vi "image recorder main panel.vi"() -> ()   [LabVIEW 2013]
uses:
  <vilib>/Utility/error.llb/DialogType.ctl
  Image-Stack-Compressor/StackWriterWrapper/LV code/StackWriterWrapper.lvlib
  <vilib>/ptbypt/NI_PtbyPt.lvlib
panel:
  out "frame add time":u32
  out "last loop time":u32
  in  "left of screen":string="air inlet"
  in  "bottom of screen":string="CS"
  in  "top of screen":string="back of box (y = 0)"
  in  "central region (frac)":dbl caption="central region for placement\nsize (fraction of full screen)"
  out "loop time":u32
  in  "max Background Compression Threads":i32=4
  in  "maxBytesToWrite":u64=1950000000 format="%.2p"
  in  "limit file size?":bool
  out "notes last updated":timestamp format="%<%I:%M %p\n%d/%m/%y>T"
  in  "notes":string
  out "avg frame rate (fps)":dbl
  out "total loop\nwith delay":u32
  out "delay time":dbl
  in  "auto-set":bool
  out "numToWrite":i32(slide) scale=0.0..10.0
  out "numToCompress":i32(slide)=1 scale=0.0..10.0
  out "loop too fast":bool
  in  "min loop time (ms)":u32
  out "timing report":string="-\n  name: adding frame to stack\n  ncalls: 72\n  totaltime: 0.298202\n  maxtime: 0.00436328\n  mintime: 0.00225001\n  avg time: 0.00414169\n  numblowntics: 0\n-\n  name: cloning image\n  ncalls: 72\n  totaltime: 0.24642\n  maxtime: 0.00378184\n  mintime: 0.0017782\n  avg time: 0.0034225\n  numblowntics: 0\n-\n  name: compressing a frame\n  ncalls: 72\n  totaltime: 1.94123\n  maxtime: 0.0403699\n  mintime: 0.0239481\n  avg time: 0.0269615\n  numblowntics: 0\n-\n  name: creating save description\n  ncalls: 1\n  totaltime: 6.19014e-005\n  maxtime: 6.19014e-005\n  mintime: 6.19014e-005\n  avg time: 6.19014e-005\n  numblowntics: 0\n-\n  name: deleting written stack from memory\n  ncalls: 1\n  totaltime: 0.00222322\n  maxtime: 0.00222322\n  mintime: 0.00222322\n  avg time: 0.00222322\n  numblowntics: 0\n-\n  name: writing a stack to disk\n  ncalls: 1\n  totaltime: 0.0259505\n  maxtime: 0.0259505\n  mintime: 0.0259505\n  avg time: 0.0259505\n  numblowntics: 0\ncxcore: 1.0.0, cv: 1.0.0\n\n"
  out "stack destination":string="C:\\data\\test\\t10\\n#n#n#n\\CS(CS)\\2011\\09\\14\\1334\\CS@CS@t10@n#n#n#n@30.mmf"
  out "stackwriter pointer":u32=314603384
  out "loop iteration":i32=23494
  out "error out":errorcluster
  out "maximum loop time":u32
  out "average loop time":dbl format="%.2p"
  in  "max stack size":dbl=1.99
  out "GB written":dbl format="%.2f"
  out "max file size in GB":u64=8589934591
  out "MB written":i32
  out "average time to compress a frame":dbl format="%#_3p"
  out "average time to add a frame to stack":dbl format="%#_3p"
  out "average time to write a stack":dbl format="%#_3p"
  out "elapsed time(s)":dbl
  in  "anticipated frame rate":dbl=30.0
  in  "lgDimMinSize":i32=5
  in  "keyFrameInterval":i32=90
  in  "smallDimMinSize":i32=3
  in  "thresholdAboveBackground":i32=7
  out "buffer number":u32
  in  "base directory":path=path "C:/data/test"
  out "filename":string="CS@CS@t10@n#n#n#n@30"
  out "data directory":path=path "C:/data/test/t10/n#n#n#n/CS(CS)/2011/09/14/1334"
  in  "setup camera?":bool
  in  "STOP PROGRAM":bool
  in  "STOP ACQUISITION":bool
  in  "MAKE DIRECTORIES":bool
  in  "START ACQUISITION":bool
  in  "use ROI":bool
  in  "region of interest":cluster{"x0":u32, "y0":u32, "w":u32, "h":u32}={"x0"=0, "y0"=0, "w"=5000, "h"=5000}
  in  "Acquisiton Time (s)":dbl=660.0
  in  "update image every __ ms":u16=500
  out "Camera Image":T1(plugin-control)
  in  "set all control values as default":bool
  out "GAL4 Line":string="CS"
  in  "Experiment Description":T2={"GAL4 Line / Line A / Genotype"="CS", "UAS-Effector Line / Line B"="", "Experiment Type"=enum."olfaction", "Stimulus Descriptions"=[{"Stimulus Modulation"=enum."Spatial", "stimulant"="co2", "hi"=5, "lo"=0, "period"=20, "Modulation Detail"=enum."LinearX", "unit"="pct", "period_unit"="cm", "additional description"=enum."none", "description"=""}], "other name"="", "Training/Habituation Pre Exposure"={"CS"="", "UCS"="", "Training Protocol"="", "Training ID Code"="", "Training Type"=enum."none (no directory)"}}
  # "MMF compression settings"
  # "to reset to actual defaults, delete file\nimage recorder main panel ctl values.dflt"
  # "debugging stuff"
  # "X"
  # "lady gaga convention: when gradient is forward odor 1 \nhas minimum in lo field and maximum in hi field"
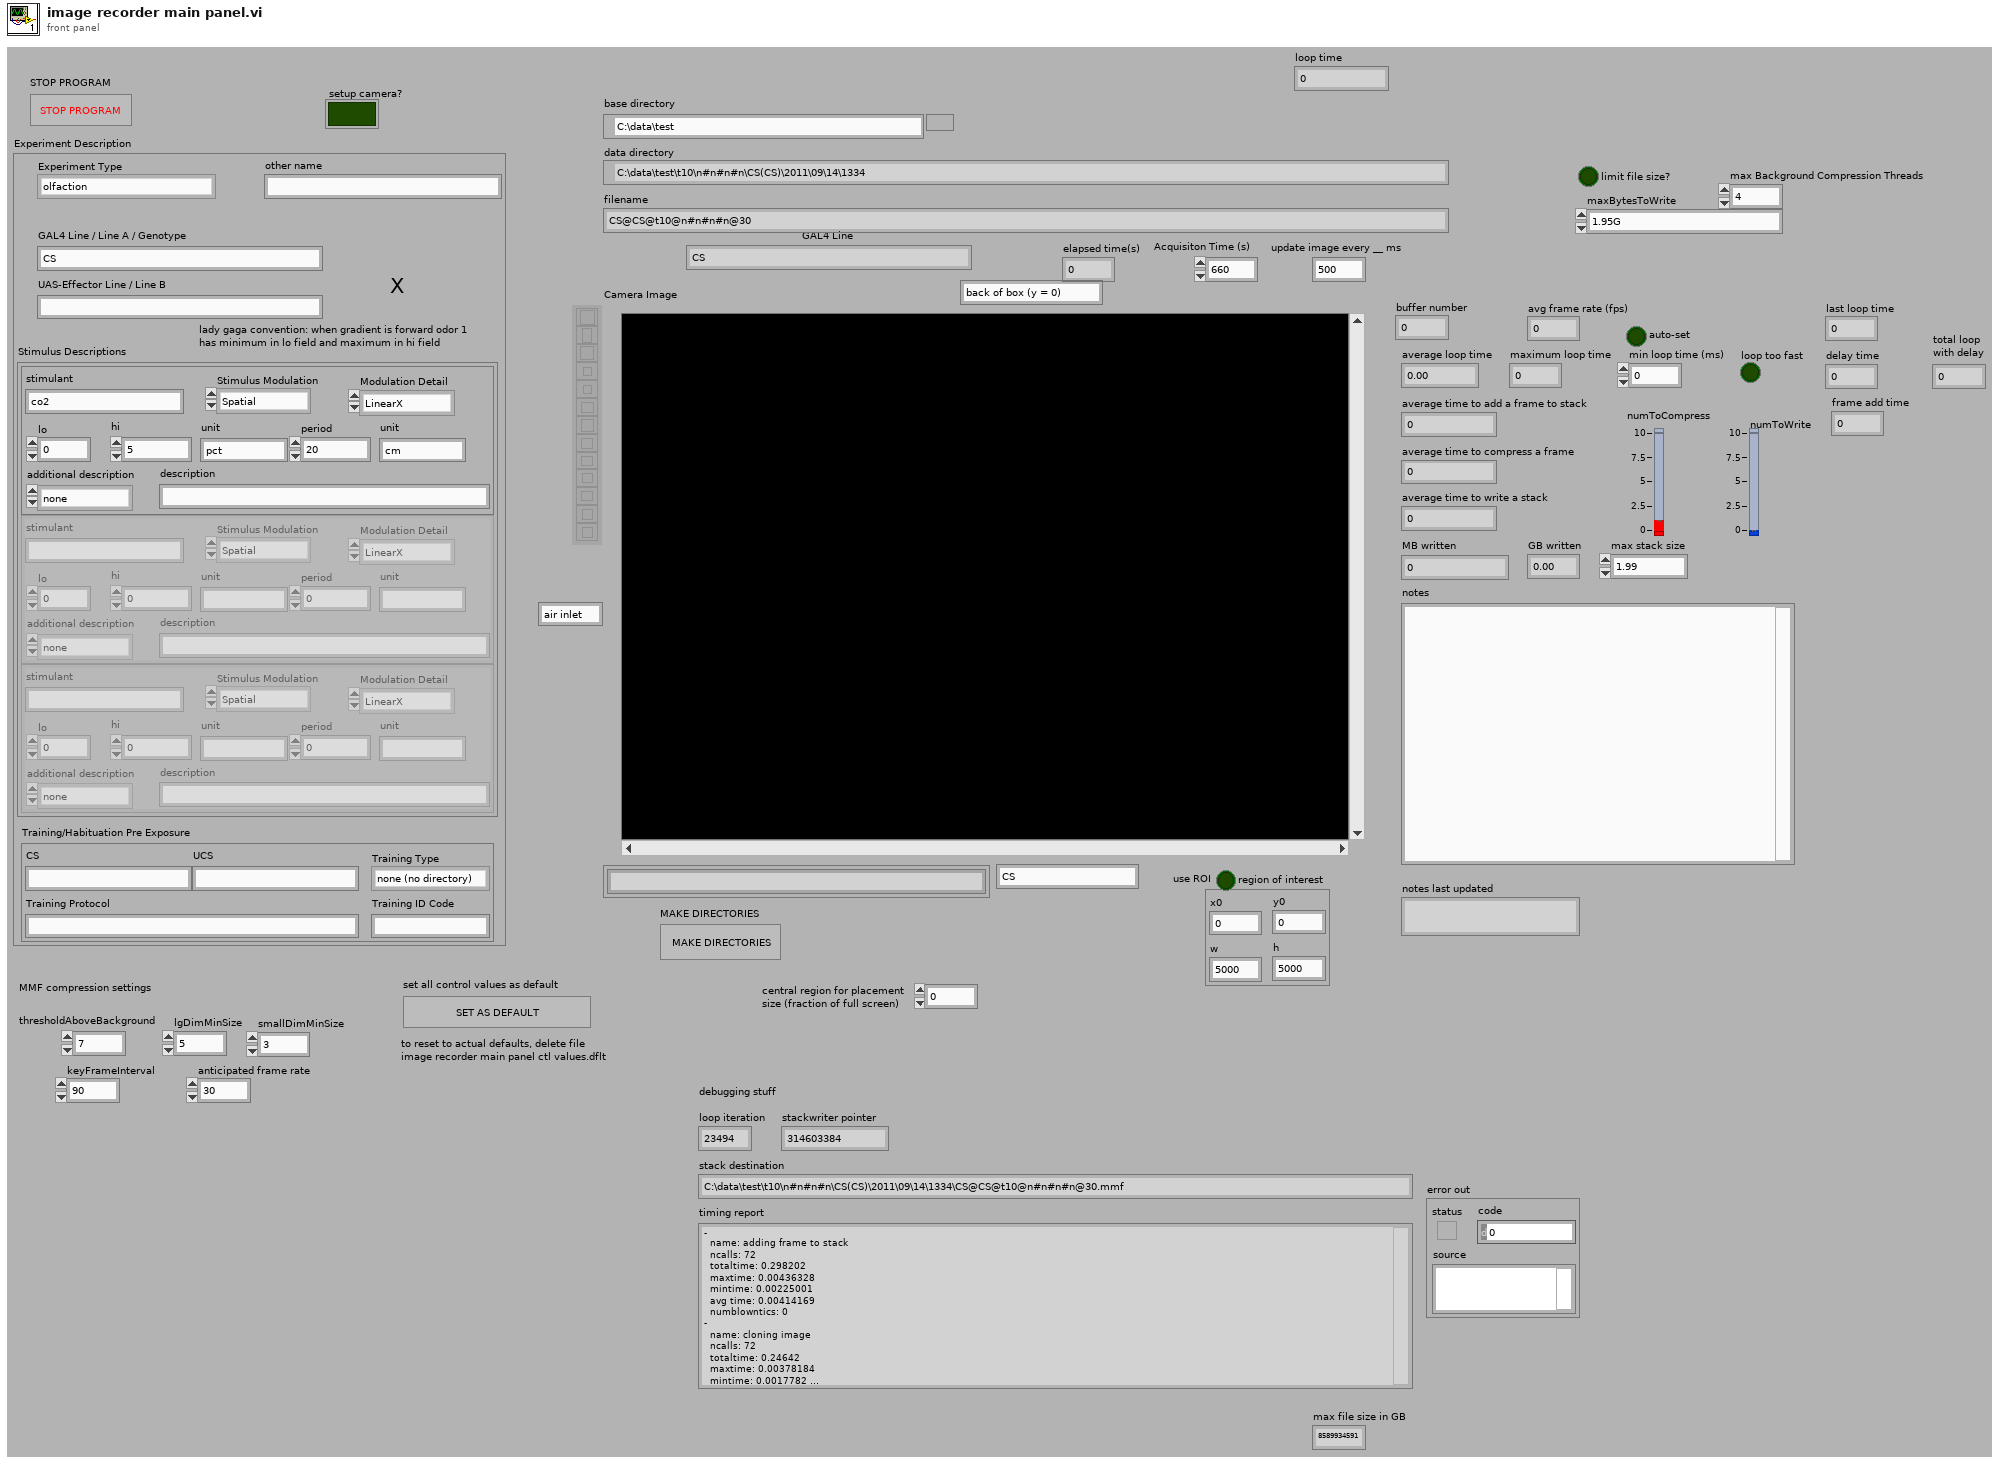
[diagram p1: front panel]
types:
  T1 = typedef "IMAQ Image.ctl" = refnum<image>
  T2 = cluster{"GAL4 Line / Line A / Genotype":string, "UAS-Effector Line / Line B":string, "Experiment Type":enum16{"other", "olfaction", "phototaxis", "chemotaxis", "thermotaxis", "multi sensory"}, "Stimulus Descriptions":cluster{"Stimulus Modulation":enum16{"Spatial", "Temporal", "Constant", "Other"}, "stimulant":string, "hi":u16, "lo":u16, "period":u16, "Modulation Detail":enum16{"LinearX", "LinearY", "Triangle", "Sine", "Square", "AngledX", "AngledY"}, "unit":string, "period_unit":string, "additional description":enum16{"none", "append", "replace"}, "description":string}[], "other name":string, "Training/Habituation Pre Exposure":cluster{"CS":string, "UCS":string, "Training Protocol":string, "Training ID Code":string, "Training Type":enum16{"none (no directory)", "untrained", "trained"}}}
  T3 = typedef "DialogType.ctl" = u16
  T4 = typedef "IMAQdx.ctl" = refnum<k21>
  T5 = cluster{"Aquisition Type":enum16{"IMAQ", "IMAQdx", "AVI", "MMF", "STACK"}, "Interface Name":string, "use roi":bool, "ROI":cluster{"left":u16, "top":u16, "width":u16, "height":u16}, "camera name":T4, "AVI Path":path, "mmf path":path, "stub":string, "Field Width (0 disables 0 padding)":u8, "extension":string, "inter-frame interval (ms)":dbl}
  T6 = typedef "AviRefnum.ctl" = refnum<k1>
  T7 = cluster{"Aquisition Type":enum16{"IMAQ", "IMAQdx", "AVI", "MMF", "STACK"}, "IMAQ Session Out":refnum<k11>, "imaqdx session":T4, "AVI parameters":cluster{"Avi Refnum ":T6, "inter-frame interval (ms)":dbl}, "mmf parameters":cluster{"mmf pointer":u32, "inter-frame interval (ms)":dbl}, "stack read info":cluster{"file stub":string, "format string":string, "extension":string, "inter-frame interval (ms)":dbl}, "camera image":T1, "camera image is 8 bit":bool, "8 bit camera image":T1}
  T8 = enum16{"Reset Table", "Get Values", "Add Value", "Get Table", "Get Spreadsheet", "set stack writer"}
  T9 = enum16{"open", "replace", "create", "open or create", "replace or create", "replace or create with confirmation"}
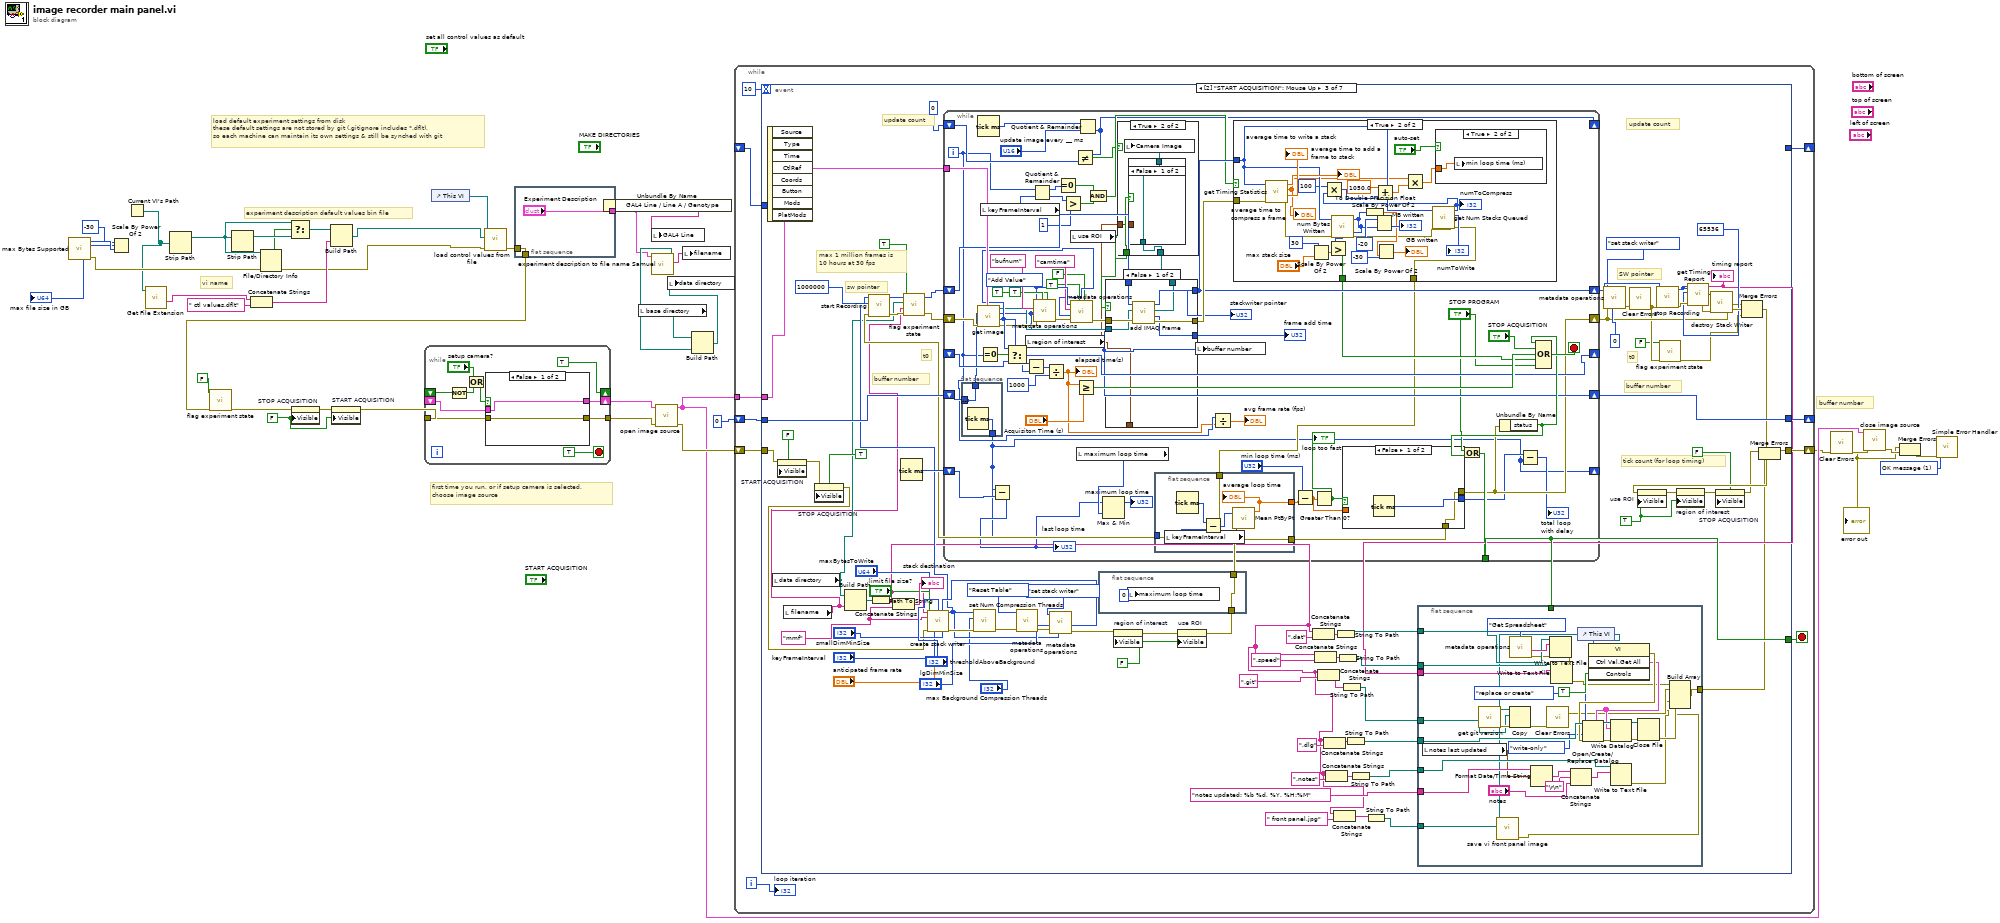
[diagram p0: block diagram]
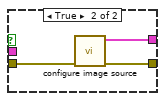
[diagram p2: hidden frame]
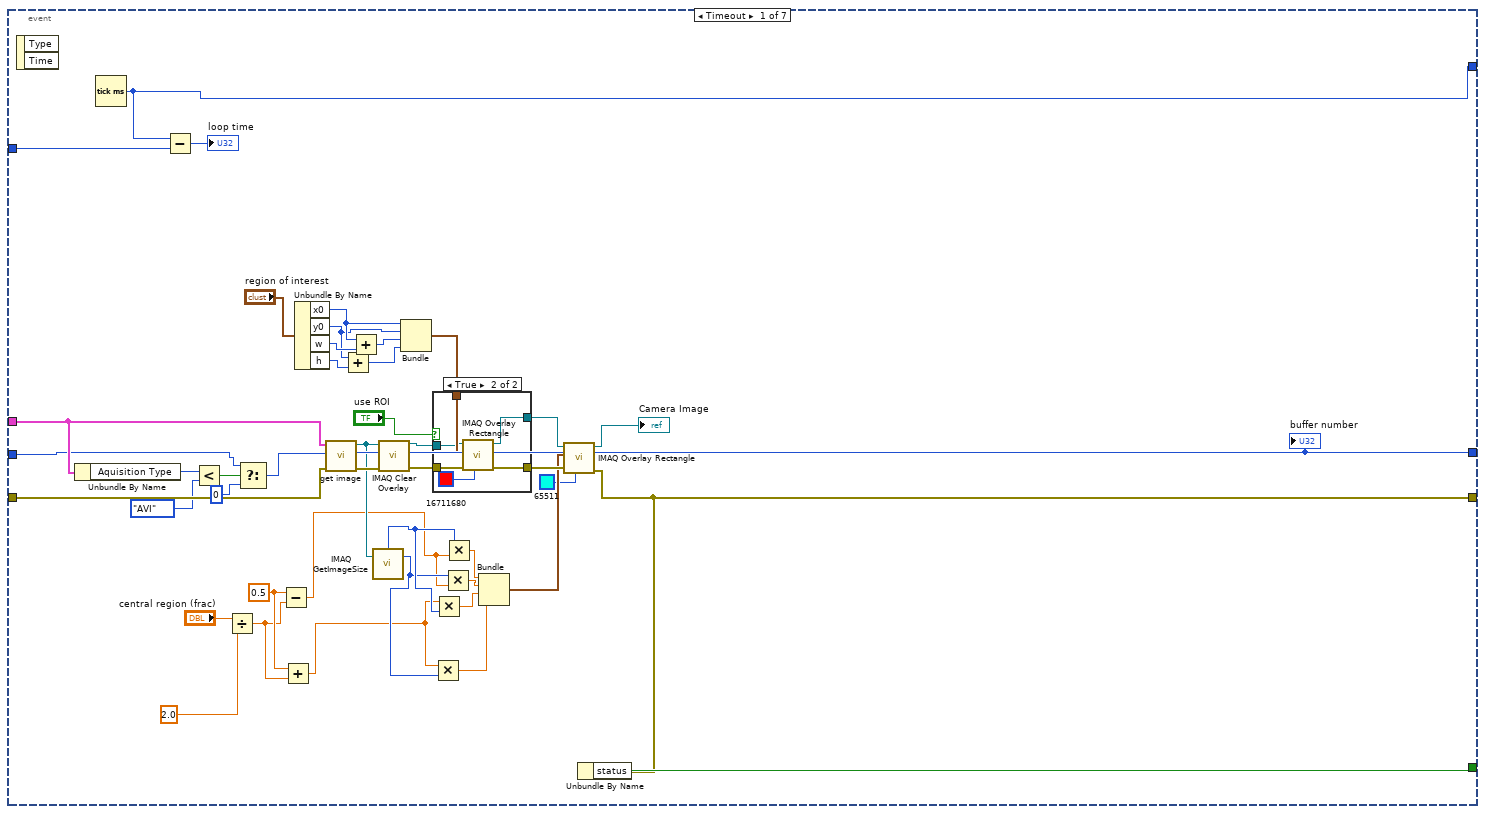
[diagram p3: hidden frame]
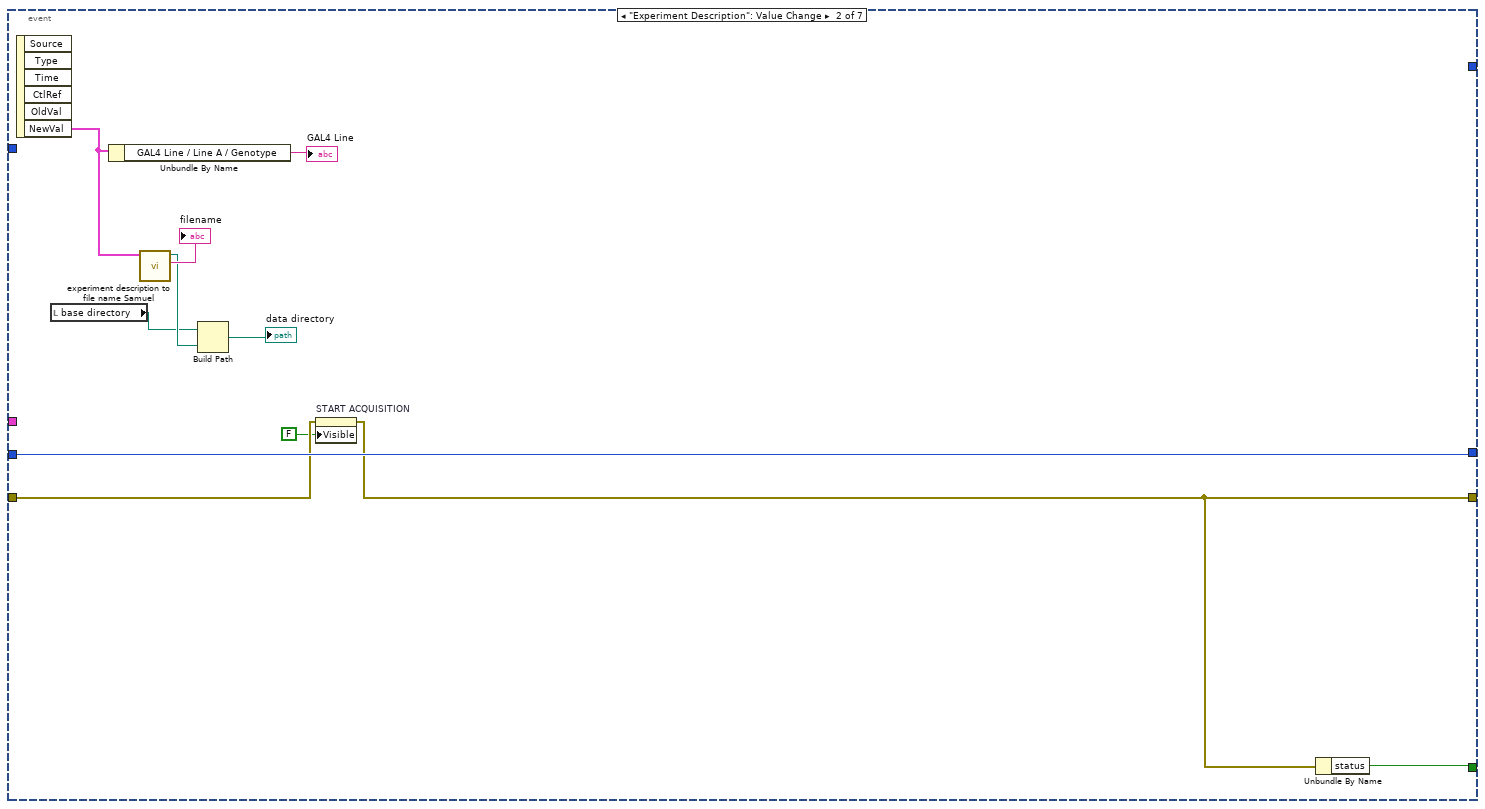
[diagram p5: hidden frame]
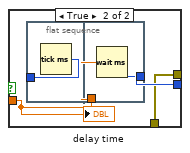
[diagram p6: hidden frame]
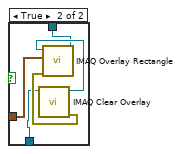
[diagram p8: hidden frame]
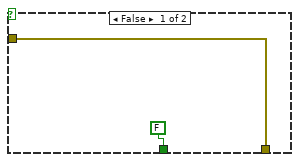
[diagram p9: hidden frame]
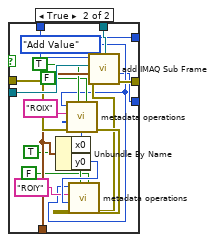
[diagram p11: hidden frame]
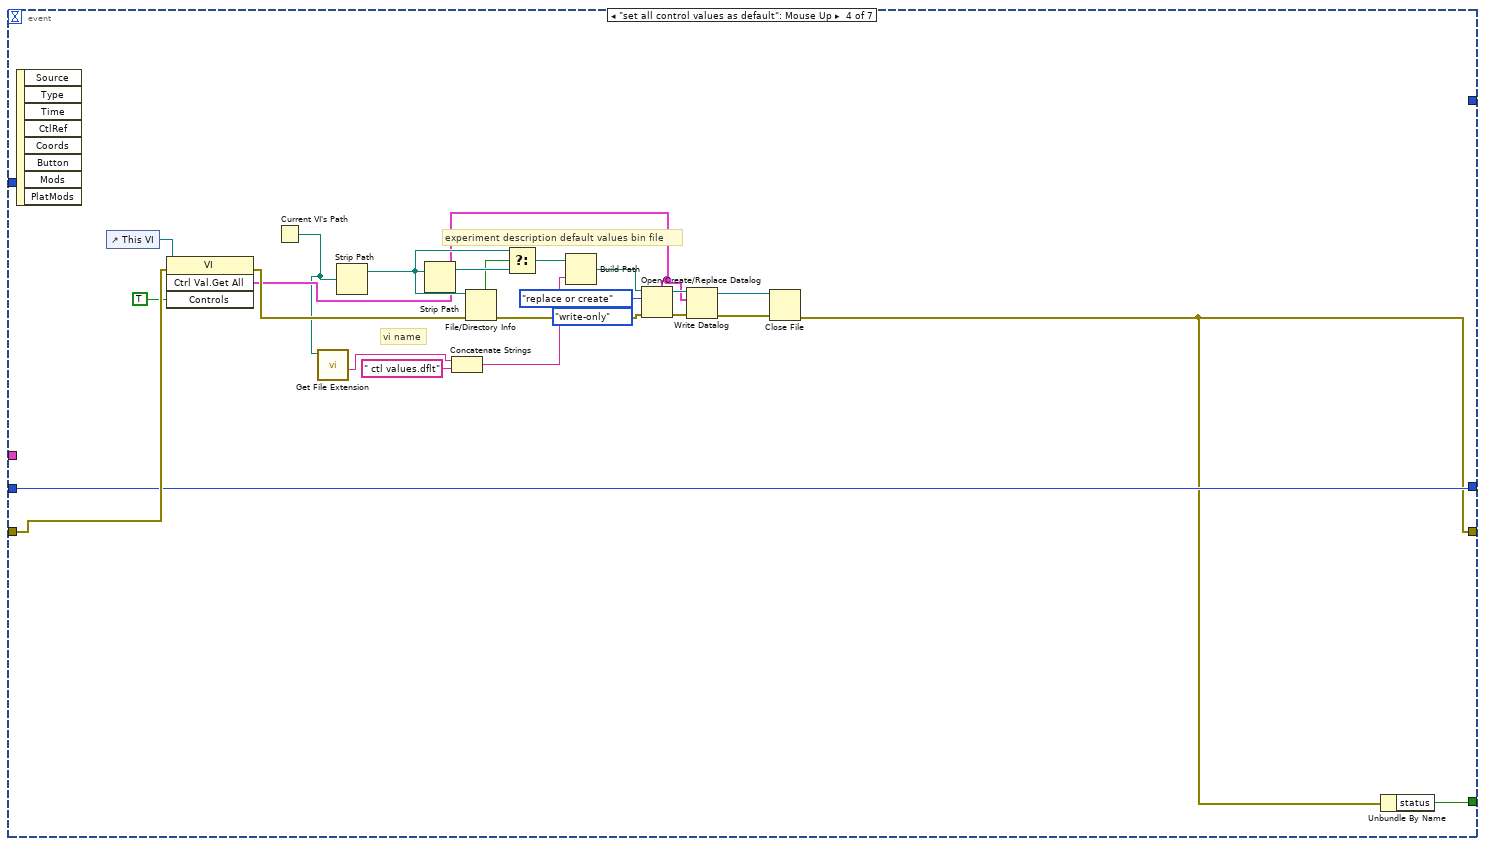
[diagram p12: hidden frame]
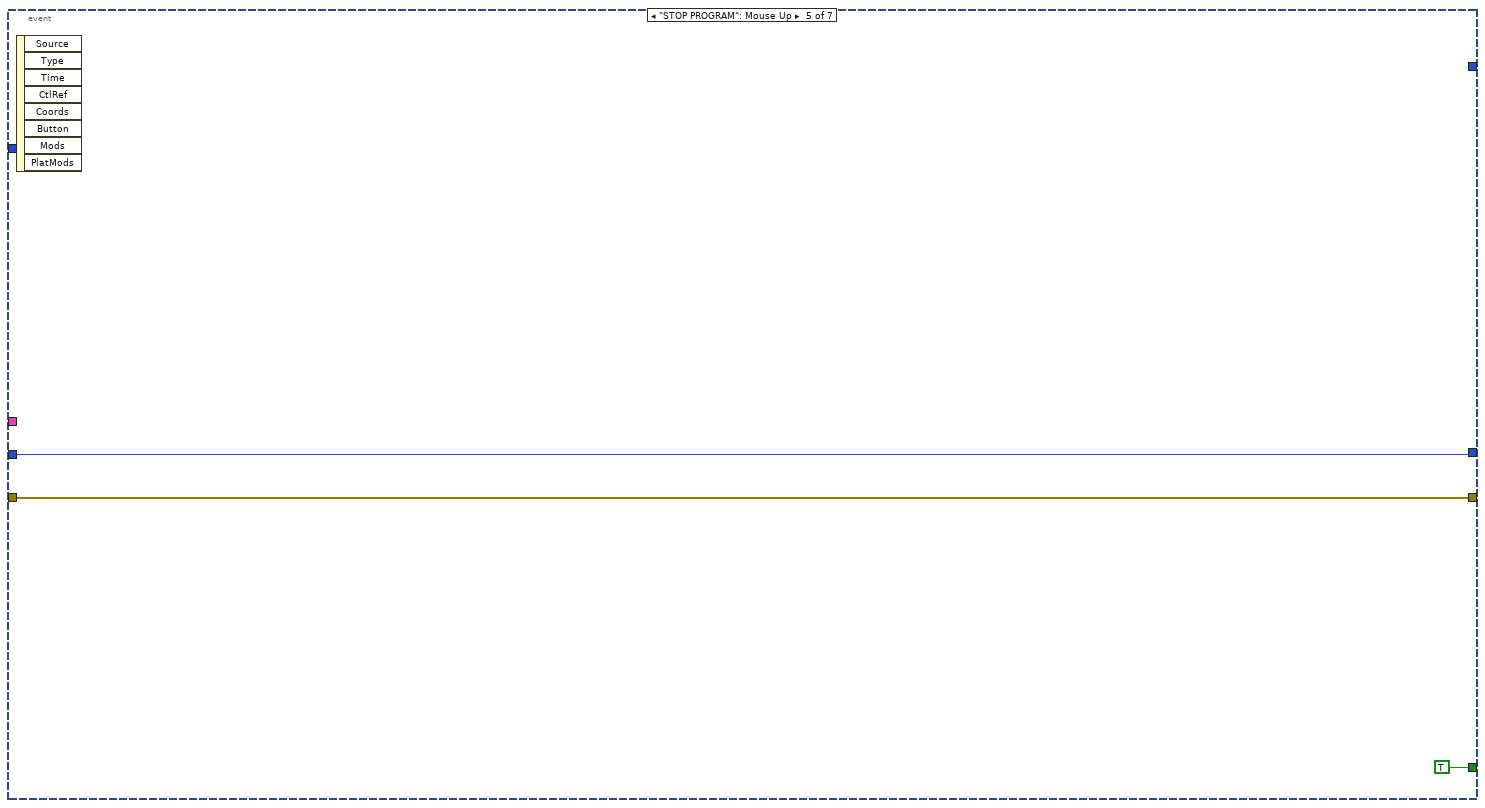
[diagram p13: hidden frame]
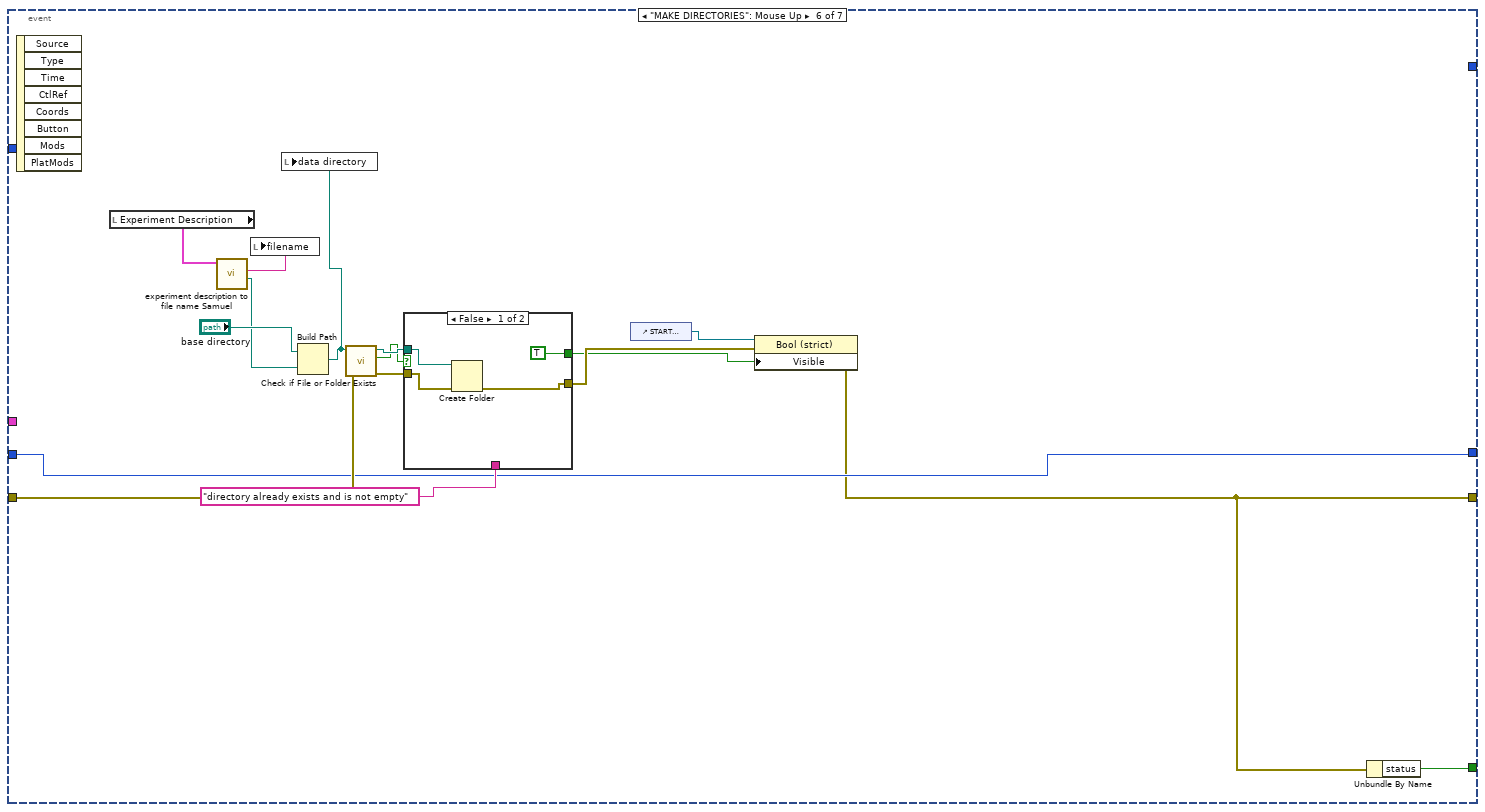
[diagram p14: hidden frame]
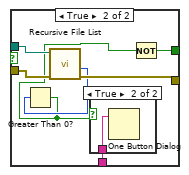
[diagram p15: hidden frame]
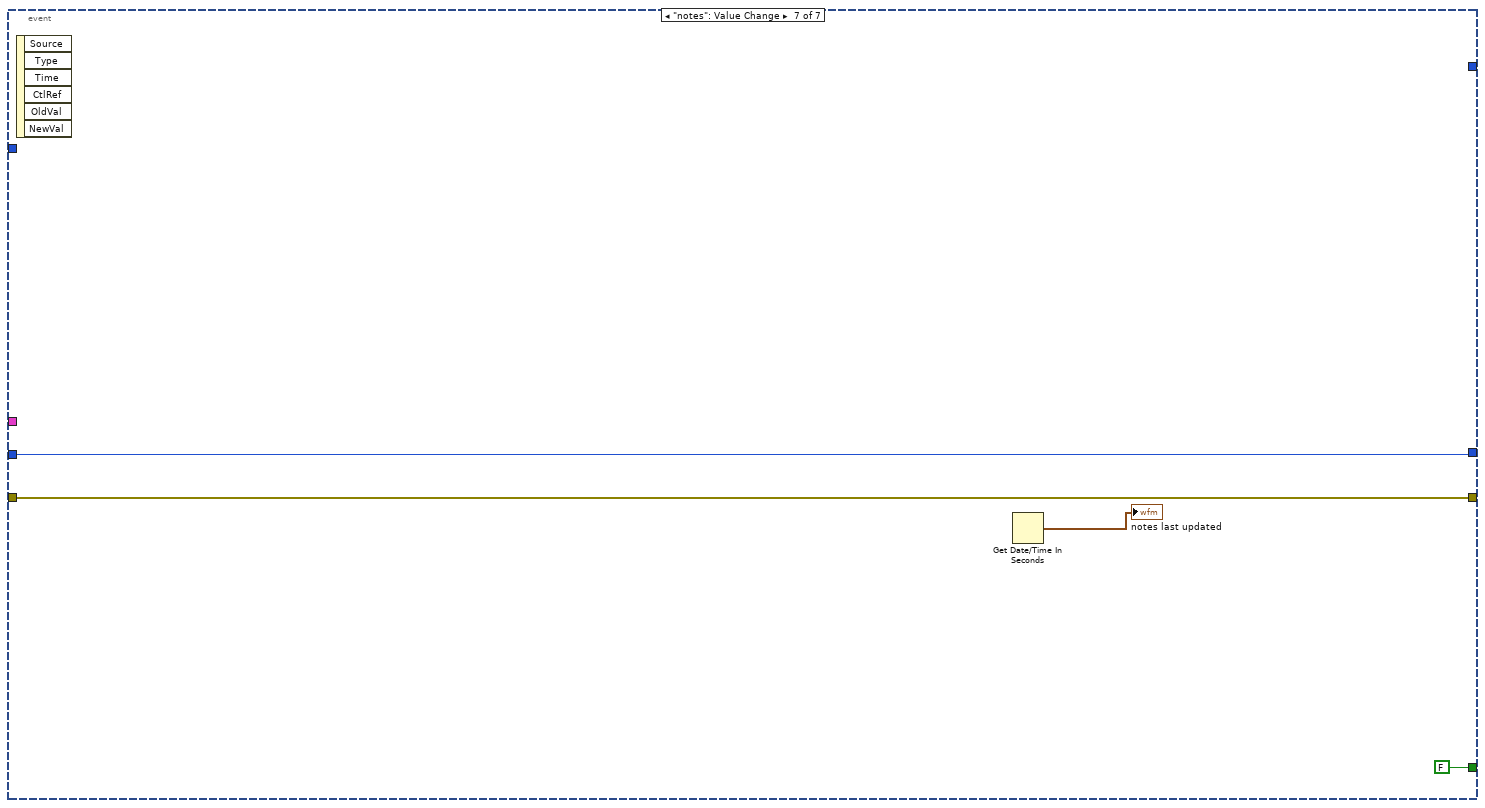
[diagram p17: hidden frame]
diagram:
  w14 = T3 1 items=["no dialog", "OK message", "continue or stop message", "OK message + warnings", "continue/stop + warnings"] ("type of dialog (OK msg:1)")
  w26 = FALSE ("Visible")
  # "buffer number"
  # "first time you run, or if setup camera is selected, \nchoose image source"
  # "load default experiment settings from disk\nthese default settings are not stored by git (.gitignore includes *.dflt), \nso each machine can maintain its own settings & still be synched with git"
  # "experiment description default values bin file"
  # "vi name"
  n1 = call "max Bytes Supported.vi"() -> ("error out"=w23:errorcluster, "function return"=w22:u32)  [unwired: 10 in]
  n2 = Scale By Power Of 2(n=-30, x=w22) -> (x*2^n=→"max file size in GB":u32)
  n3 = Current VI's Path() -> (path=w4:path)
  n4 = call <vilib>:"Get File Extension.vi"("file"=w4) -> ("filename without extension"=w3:string)  [unwired: 7 in, 3 out]
  n5 = Strip Path(path=w4) -> (stripped path=w38:path)  [unwired: 1 out]
  n6 = call "flag experiment state.vi"("error in (no error)"=w7, "experiment started"=FALSE) -> ("error out"=w2:errorcluster)  [unwired: 9 in]
  n7 = Strip Path(path=w38) -> (stripped path=w37:path)  [unwired: 1 out]
  n8 = Concatenate Strings(w3, " ctl values.dflt" ("string")) -> (w33:string)
  n9 = File/Directory Info(path=w38, error in=w23) -> (directory=w36:bool, error out=w10:errorcluster)  [unwired: 5 out]
  n10 = Select(t=w38, s=w36, f=w37) -> (s? t:f=w34:path)
  n11 = property on="STOP ACQUISITION" class="Bool"(error in=w2, "Visible"=w26) -> (error out=w27:errorcluster)  [unwired: 1 in, 1 out]
  n12 = Build Path(base path=w34, name or relative path=w33) -> (appended path=w9:path)
  n13 = property on="START ACQUISITION" class="Bool (strict)"(error in=w27, "Visible"=w26) -> (error out=w25:errorcluster)  [unwired: 1 in, 1 out]
  n14 = while {
    shift-right: [TRUE] -> _
    shift-left: _ -> [w44]
    tunnel: w25 -> [w42]
    tunnel: [w41] -> w30
    shift-right: [w40] -> w31
    shift-left: _ -> [w39]
    stop <- TRUE stop-if-true
    n15 = Not(x=w44) -> (.not. x?=w43:bool)
    n16 = Or(x="setup camera?", y=w43) -> (x .or. y?=w46:bool)
    n17 = case shown="False" w46 {
      tunnel: w42 -> [w49 w53]
      tunnel: [w49 w52] -> w41
      tunnel: [w50 w51] -> w40
      tunnel: w39 -> [w50 _]
      frame False {
      }
      frame True {
        n18 = call "configure image source.vi"("error in (no error)"=w53) -> ("error out"=w52:errorcluster, "image source parameters"=w51:T5)  [unwired: 9 in]
      }
    }
  }
  n19 = control-ref of="This VI"() -> (w5:refnum<vi>)
  n20 = call "load control values from file.vi"("error in (no error)"=w10, "datalog path (use dialog)"=w9, "VI ref"=w5) -> ("error out"=w8:errorcluster)  [unwired: 8 in]
  n21 = flat-sequence {
    tunnel: w8 -> [w55]
    tunnel: [w55] -> w7
    tunnel: ["Experiment Description"] -> w6
    frame #0 {
    }
  }
  n22 = Unbundle By Name(w6) -> ("GAL4 Line / Line A / Genotype"=w32:string)
  n23 = local read "base directory"() -> (w13:path)
  n24 = local write "GAL4 Line"(w32) -> ()
  n25 = call "experiment description to file name Samuel.vi"("Experiment Description"=w6) -> ("filename"=w24:string, "data directory"=w12:path)  [unwired: 8 in, 1 out]
  n26 = call "open image source.vi"("error in (no error)"=w30, "image source parameters"=w31) -> ("error out"=w29:errorcluster, "image source data"=w19:T7)  [unwired: 8 in]
  n27 = local write "filename"(w24) -> ()
  n28 = Build Path(base path=w13, name or relative path=w12) -> (appended path=w11:path)
  n29 = local write "data directory"(w11) -> ()
  n30 = while {
    shift-right: [w61] -> w16
    shift-left: w29 -> [w64]
    tunnel: w19 -> [w63]
    shift-right: [w60] -> _
    shift-left: 0 -> [w62]
    shift-right: [w57] -> _
    shift-left: _ -> [w56]
    i -> [w59]
    stop <- w65 stop-if-true
    n31 = event shown="[2] \"START ACQUISITION\": Mouse Up" {
      selector: _ -> [_ _ _ _ _ _ _]
      dyn-events: _ -> [_ _ _ _ _ _ _]
      timeout: 10 -> [_ _ _ _ _ _ _]
      tunnel: [w100 w126 w173 w398 TRUE ("status") w425 FALSE ("status")] -> w65
      tunnel: w64 -> [w109 w123 w197 w418 w420 w436 w452]
      tunnel: w63 -> [w108 _ w201 _ _ _ _]
      tunnel: w62 -> [w104 w127 w203 w400 w422 w426 w451]
      tunnel: [w83 w121 w156 w399 w420 w424 w452] -> w61
      tunnel: [w101 w127 w202 w400 w422 w426 w451] -> w60
      tunnel: [w86 _ _ _ _ _ _] -> w57
      tunnel: w56 -> [w87 _ _ _ _ _ _]
      event Timeout {
        w71 = 0.5 ("x")
        n32 = event-data() -> ()  [unwired: 1 in, 2 out]
        n33 = Unbundle By Name(w108) -> ("Aquisition Type"=w107:enum16{"IMAQ", "IMAQdx", "AVI", "MMF", "STACK"})
        n34 = Tick Count (ms)() -> (millisecond timer value=w86:u32)
        n35 = Subtract(x=w86, y=w87) -> (x-y=→"loop time":u32)
        n36 = Less?(x=w107, y=enum16{"IMAQ", "IMAQdx", "AVI", "MMF", "STACK"}."AVI") -> (x < y?=w105:bool)
        n37 = Divide(x="central region (frac)", y=2.0) -> (x/y=w68:dbl)
        n38 = Select(t=w104, s=w105, f=0) -> (s? t:f=w102:u32)
        n39 = Subtract(x=w71, y=w68) -> (x-y=w67:dbl)
        n40 = Add(x=w71, y=w68) -> (x+y=w66:dbl)
        n41 = Unbundle By Name("region of interest") -> ("x0"=w94:u32, "y0"=w93:u32, "w"=w96:u32, "h"=w95:u32)
        n42 = call "get image.vi"("error in (no error)"=w109, "previous buffer number"=w102, "image source data"=w108) -> ("error out"=w99:errorcluster, "buffer number"=w101:u32, "captured image"=w80:T1)  [unwired: 5 in, 1 out]
        "buffer number" <- w101
        n43 = Add(x=w93, y=w95) -> (x+y=w91:u32)
        n44 = Add(x=w94, y=w96) -> (x+y=w92:u32)
        n45 = call "IMAQ GetImageSize"("Image"=w80) -> ("Y Resolution"=w76:i32, "X Resolution"=w77:i32)  [unwired: 3 in, 1 out]
        n46 = call "IMAQ Clear Overlay"("error in (no error)"=w99, "Image"=w80) -> ("error out"=w88:errorcluster, "Image Out"=w89:T1)  [unwired: 8 in]
        n47 = Bundle("x0"=w94, "y0"=w93, w92, w91) -> (w90:cluster{"x0":u32, "y0":u32, u32, u32})  [unwired: 1 in]
        n48 = case shown="True" "use ROI" {
          tunnel: w90 -> [_ w117]
          tunnel: w89 -> [w111 w116]
          tunnel: w88 -> [w110 w115]
          tunnel: [w111 w113] -> w81
          tunnel: [w110 w112] -> w84
          frame False {
          }
          frame True {
            n49 = call "IMAQ Overlay Rectangle"("Color"=u32 16711680, "error in (no error)"=w115, "Rectangle"=w117, "Image"=w116) -> ("error out"=w112:errorcluster, "Image Out"=w113:T1)  [unwired: 6 in]
          }
        }
        n50 = Multiply(x=w66, y=w76) -> (x*y=w74:dbl)
        n51 = Multiply(x=w66, y=w77) -> (x*y=w75:dbl)
        n52 = Multiply(x=w76, y=w67) -> (x*y=w78:dbl)
        n53 = Multiply(x=w77, y=w67) -> (x*y=w79:dbl)
        n54 = Bundle(w79, w78, w75, w74) -> (w73:cluster{dbl, dbl, dbl, dbl})  [unwired: 1 in]
        n55 = call "IMAQ Overlay Rectangle"("Color"=u32 65511, "error in (no error)"=w84, "Rectangle"=w73, "Image"=w81) -> ("error out"=w83:errorcluster, "Image Out"=→"Camera Image":T1)  [unwired: 6 in]
        n56 = Unbundle By Name(w83) -> ("status"=w100:bool)
      }
      event "Experiment Description": Value Change {
        n57 = event-data() -> ("NewVal"=w125:T2)  [unwired: 1 in, 5 out]
        n58 = local read "base directory"() -> (w119:path)
        n59 = Unbundle By Name(w125) -> ("GAL4 Line / Line A / Genotype"=→"GAL4 Line":string)
        n60 = call "experiment description to file name Samuel.vi"("Experiment Description"=w125) -> ("filename"=→"filename":string, "data directory"=w120:path)  [unwired: 8 in, 1 out]
        n61 = Build Path(base path=w119, name or relative path=w120) -> (appended path=→"data directory":path)
        n62 = property on="START ACQUISITION" class="Bool (strict)"(error in=w123, "Visible"=FALSE) -> (error out=w121:errorcluster)  [unwired: 1 in, 1 out]
        n63 = Unbundle By Name(w121) -> ("status"=w126:bool)
      }
      event "START ACQUISITION": Mouse Up {
        w179 = TRUE ("Visible")
        w189 = FALSE ("Visible")
        w140 = "mmf" ("string")
        # "tick count (for loop timing)"
        # "max 1 million frames is \n10 hours at 30 fps"
        # "update count"
        # "buffer number"
        # "t0"
        # "update count"
        # "sw pointer"
        # "buffer number"
        # "t0"
        # "SW pointer"
        n64 = event-data() -> ()  [unwired: 1 in, 8 out]
        n65 = local read "data directory"() -> (w134:path)
        n66 = property on="START ACQUISITION" class="Bool (strict)"(error in=w197, "Visible"=FALSE) -> (error out=w199:errorcluster)  [unwired: 1 in, 1 out]
        n67 = local read "filename"() -> (w133:string)
        n68 = property on="STOP ACQUISITION" class="Bool"(error in=w199, "Visible"=TRUE) -> (error out=w196:errorcluster)  [unwired: 1 in, 1 out]
        n69 = Build Path(base path=w134, name or relative path=w133) -> (appended path=w210:path)
        n70 = Path To String(path=w210) -> (string=w132:string)
        n71 = Concatenate Strings(w132, w140) -> (→"stack destination":string)
        n72 = Tick Count (ms)() -> (millisecond timer value=w183:u32)
        n73 = call "create stack writer.vi"("file stub"=w132, "keyFrameInterval"="keyFrameInterval", "thresholdAboveBackground"="thresholdAboveBackground", "lgDimMinSize"="lgDimMinSize", "extension"=w140, "limit file size?"="limit file size?", "maxBytesToWrite"="maxBytesToWrite", "error in (no error)"=w196, "anticipated frame rate"="anticipated frame rate", "smallDimMinSize"="smallDimMinSize") -> ("stack writer pointer"=w136:u32, "error out"=w192:errorcluster)  [unwired: 4 in]
        n74 = call "start Recording.vi"("error in (no error)"=w181, "nframes"=1000000, "sw"=w136) -> ("error out"=w187:errorcluster, "sw out"=w188:u32)  [unwired: 6 in, 1 out]
        n75 = call "flag experiment state.vi"("error in (no error)"=w187, "filename"=w133, "data directory"=w134, "experiment started"=TRUE) -> ("error out"=w145:errorcluster)  [unwired: 7 in]
        n76 = while {
          shift-right: [w293] -> w150
          shift-left: w188 -> [w297]
          shift-right: [w262] -> w147
          shift-left: w145 -> [w314]
          shift-right: [w270] -> w202
          shift-left: w203 -> [w263]
          shift-right: [w271] -> _
          shift-left: _ -> [w311]
          tunnel: w201 -> [w313]
          shift-right: [w276] -> _
          shift-left: u32 0 -> [w295]
          tunnel: [w285] -> w173
          shift-right: [w251] -> _
          shift-left: w183 -> [w274]
          i -> [w257]
          stop <- w289 stop-if-true
          w306 = T8."Add Value" ("Operation")
          n77 = flat-sequence {
            tunnel: [w322] -> w251
            tunnel: [w321] -> w264
            tunnel: [w321] -> _
            tunnel: w263 -> [w321]
            frame #0 {
              n78 = Tick Count (ms)() -> (millisecond timer value=w322:u32)
            }
          }
          n79 = Tick Count (ms)() -> (millisecond timer value=w288:u32)
          n80 = call "get image.vi"("error in (no error)"=w314, "previous buffer number"=w264, "image source data"=w313) -> ("error out"=w303:errorcluster, "aquisition time ms"=w304:u32, "buffer number"=w270:u32, "captured image"=w298:T1)  [unwired: 5 in]
          n81 = Equal To 0?(x=w257) -> (x = 0?=w312:bool)
          n82 = local read "keyFrameInterval"() -> (w284:i32)
          n83 = Subtract(x=w251, y=w274) -> (x-y=w254:u32)
          "last loop time" <- w254
          n84 = Select(t=w304, s=w312, f=w311) -> (s? t:f=w271:u32)
          n85 = local read "region of interest"() -> (w258:cluster{"x0":u32, "y0":u32, "w":u32, "h":u32})
          n86 = Subtract(x=w304, y=w271) -> (x-y=w296:u32)
          n87 = Quotient & Remainder(x=w257, y=w284) -> (x-y*floor(x/y)=w283:i32, floor(x/y)=w282:i32)
          n88 = call "metadata operations.vi"("add time?"=TRUE, "add to stack writer"=TRUE, "error in (no error)"=w303, "value"=w270, "key"="bufnum", "Operation"=w306) -> ("error out"=w302:errorcluster)  [unwired: 2 in, 3 out]
          n89 = Divide(x=w296, y=u32 1000) -> (x/y=w256:dbl)
          "elapsed time(s)" <- w256
          n90 = Equal To 0?(x=w283) -> (x = 0?=w280:bool)
          n91 = Greater?(x=w282, y=1) -> (0:w279:bool)
          n92 = local read "use ROI"() -> (w259:bool)
          n93 = call "metadata operations.vi"("add time?"=FALSE, "add to stack writer"=TRUE, "error in (no error)"=w302, "value"=w304, "key"="camtime", "Operation"=w306) -> ("error out"=w299:errorcluster)  [unwired: 2 in, 3 out]
          n94 = Greater Or Equal?(x=w256, y="Acquisiton Time (s)") -> (x >= y?=w290:bool)
          n95 = local read "maximum loop time"() -> (w272:u32)
          n96 = Quotient & Remainder(x=w288, y="update image every __ ms") -> (floor(x/y)=w276:u32)  [unwired: 1 out]
          n97 = Not Equal?(x=w276, y=w295) -> (x != y?=w277:bool)
          n98 = And(x=w280, y=w279) -> (x .and. y?=w278:bool)
          n99 = Max & Min(x=w254, y=w272) -> (max(x,y)=→"maximum loop time":u32)  [unwired: 1 out]
          n100 = case shown="False" w259 {
            tunnel: w299 -> [w376 w390]
            tunnel: w298 -> [w375 w394]
            tunnel: w297 -> [w374 w395]
            tunnel: w258 -> [_ w389]
            tunnel: [w373 w393] -> w294
            tunnel: [w372 w391] -> w293
            tunnel: [w371 w392] -> w275
            tunnel: [w370 w377] -> w249
            frame False {
              n101 = call "add IMAQ Frame.vi"("error in (no error)"=w376, "Frame (8 bit 1 channel)"=w375, "Stack Writer In"=w374) -> ("error out"=w373:errorcluster, "frame add time"=w370:u32, "Frame Out"=w371:T1, "Stack Writer Out"=w372:u32)  [unwired: 5 in]
            }
            frame True {
              w378 = T8."Add Value" ("Operation")
              n102 = Unbundle By Name(w389) -> ("x0"=w383:u32, "y0"=w384:u32)
              n103 = call "metadata operations.vi"("add time?"=FALSE, "add to stack writer"=TRUE, "error in (no error)"=w390, "value"=w383, "key"="ROIX", "Operation"=w378) -> ("error out"=w386:errorcluster)  [unwired: 2 in, 3 out]
              n104 = call "metadata operations.vi"("add time?"=FALSE, "add to stack writer"=TRUE, "error in (no error)"=w386, "value"=w384, "key"="ROIY", "Operation"=w378) -> ("error out"=w385:errorcluster)  [unwired: 2 in, 3 out]
              n105 = call "add IMAQ Sub Frame.vi"("error in (no error)"=w385, "subim rectangle"=w389, "Frame (8 bit 1 channel)"=w394, "Stack Writer In"=w395) -> ("error out"=w393:errorcluster, "frame add time"=w377:u32, "Frame Out"=w392:T1, "Stack Writer Out"=w391:u32)  [unwired: 4 in]
            }
          }
          "stackwriter pointer" <- w293
          "frame add time" <- w249
          n106 = case shown="True" w277 {
            tunnel: w275 -> [_ w332]
            tunnel: w259 -> [_ w334]
            tunnel: w258 -> [_ w333]
            frame False {
            }
            frame True {
              n107 = case shown="False" w334 {
                tunnel: w333 -> [_ w340]
                tunnel: w332 -> [w335 w338]
                tunnel: [w335 w336] -> w331
                frame False {
                }
                frame True {
                  n108 = call "IMAQ Clear Overlay"("Image"=w338) -> ("error out"=w339:errorcluster, "Image Out"=w337:T1)  [unwired: 9 in]
                  n109 = call "IMAQ Overlay Rectangle"("error in (no error)"=w339, "Rectangle"=w340, "Image"=w337) -> ("Image Out"=w336:T1)  [unwired: 7 in, 1 out]
                }
              }
              n110 = local write "Camera Image"(w331) -> ()
            }
          }
          n111 = flat-sequence {
            tunnel: w253 -> [w319]
            tunnel: [w319] -> w252
            tunnel: w251 -> [w318]
            tunnel: [w316] -> w250
            frame #0 {
              n112 = local read "keyFrameInterval"() -> (w315:i32)
              n113 = Tick Count (ms)() -> (millisecond timer value=w320:u32)
              n114 = Subtract(x=w320, y=w318) -> (x-y=w317:u32)
              n115 = call <vilib>:"Mean PtByPt.vi"("x"=w317, "sample length"=w315) -> ("mean"=w316:dbl)  [unwired: 2 in, 1 out]
              "average loop time" <- w316
            }
          }
          n116 = local write "buffer number"(w270) -> ()
          n117 = Divide(x=w257, y=w256) -> (x/y=→"avg frame rate (fps)":dbl)
          n118 = case shown="True" w278 {
            tunnel: w294 -> [w341 w368]
            tunnel: w293 -> [_ w353]
            tunnel: [FALSE w357] -> w287
            tunnel: [w341 w343] -> w253
            frame False {
            }
            frame True {
              n119 = call "get Timing Statistics.vi"("error in (no error)"=w368, "sw"=w353) -> ("error out"=w367:errorcluster, "avgWriteTime"=→"average time to write a stack":dbl, "avgCompressTime"=w351:dbl, "avgAddTime"=→"average time to add a frame to stack":dbl)  [unwired: 5 in, 1 out]
              "average time to compress a frame" <- w351
              n120 = Scale By Power Of 2(n=30, x="max stack size") -> (x*2^n=w359:dbl)
              n121 = call "num Bytes Written.vi"("error in (no error)"=w367, "sw"=w353) -> ("error out"=w354:errorcluster, "function return"=w358:i32)  [unwired: 8 in]
              n122 = Greater?(x=w358, y=w359) -> (0:w357:bool)
              n123 = To Double Precision Float(number=w358) -> (double precision float=w360:dbl)
              n124 = Scale By Power Of 2(n=-20, x=w358) -> (x*2^n=→"MB written":i32)
              n125 = Scale By Power Of 2(n=-30, x=w360) -> (x*2^n=→"GB written":dbl)
              n126 = call "get Num Stacks Queued.vi"("error in (no error)"=w354, "sw"=w353) -> ("error out"=w343:errorcluster, "numToWrite"=→"numToWrite":i32, "numToCompress"=w347:i32)  [unwired: 6 in, 1 out]
              "numToCompress" <- w347
              n127 = Multiply(x=100, y=w347) -> (x*y=w345:i32)
              n128 = Add(x=1050.0 ("y"), y=w345) -> (x+y=w344:dbl)
              n129 = Multiply(x=w351, y=w344) -> (x*y=w349:dbl)
              n130 = case shown="True" "auto-set" {
                tunnel: w349 -> [_ w369]
                frame False {
                }
                frame True {
                  n131 = local write "min loop time (ms)"(w369) -> ()
                }
              }
            }
          }
          n132 = Subtract(x="min loop time (ms)", y=w250) -> (x-y=w265:dbl)
          n133 = Greater Than 0?(x=w265) -> (x > 0?=w266:bool)
          "loop too fast" <- w266
          n134 = case shown="False" w266 {
            tunnel: w265 -> [_ w327]
            tunnel: [w323 w325] -> w262
            tunnel: [w324 w326] -> w260
            tunnel: w252 -> [w323 w325]
            frame False {
              n135 = Tick Count (ms)() -> (millisecond timer value=w324:u32)
            }
            frame True {
              n136 = flat-sequence {
                tunnel: [w328] -> _
                tunnel: w327 -> [w330]
                tunnel: [w329] -> w326
                frame #0 {
                  n137 = Tick Count (ms)() -> (millisecond timer value=w328:u32)
                }
                frame #1 {
                  n138 = Wait (ms)(milliseconds to wait=w330) -> (millisecond timer value=w329:u32)
                }
              }
              "delay time" <- w327
            }
          }
          n139 = Unbundle By Name(w262) -> ("status"=w286:bool)
          n140 = Or(x="STOP PROGRAM", y=w286) -> (x .or. y?=w285:bool)
          n141 = Subtract(x=w260, y=w251) -> (x-y=→"total loop\nwith delay":u32)
          n142 = Compound Arithmetic op=OR(w286, "STOP ACQUISITION", w290, w287, "STOP PROGRAM") -> (w289:bool)
        }
        n143 = call "set Num Compression Threads.vi"("error in (no error)"=w192, "maxCompressionThreads"="max Background Compression Threads", "sw"=w136) -> ("error out"=w137:errorcluster)  [unwired: 7 in, 1 out]
        n144 = call "metadata operations.vi"("error in (no error)"=w137, "Operation"=T8."Reset Table") -> ("error out"=w193:errorcluster)  [unwired: 6 in, 3 out]
        n145 = call "metadata operations.vi"("sw"=w136, "error in (no error)"=w193, "Operation"=T8."set stack writer") -> ("error out"=w191:errorcluster)  [unwired: 5 in, 3 out]
        n146 = flat-sequence {
          tunnel: w182 -> [w247]
          tunnel: [w247] -> w181
          frame #0 {
            n147 = local write "maximum loop time"(u32 0 ("maximum loop time")) -> ()
          }
        }
        n148 = property on="region of interest" class="Clust (strict)"(error in=w191, "Visible"=w189) -> (error out=w190:errorcluster)  [unwired: 1 in, 1 out]
        n149 = property on="use ROI" class="Bool (strict)"(error in=w190, "Visible"=w189) -> (error out=w182:errorcluster)  [unwired: 1 in, 1 out]
        n150 = Concatenate Strings(w132, ".dat" ("string")) -> (w172:string)
        n151 = Concatenate Strings(w132, ".speed" ("string")) -> (w165:string)
        n152 = Concatenate Strings(w132, ".git" ("string")) -> (w161:string)
        n153 = Concatenate Strings(w132, ".dlg" ("string")) -> (w158:string)
        n154 = Concatenate Strings(w132, ".notes" ("string")) -> (w153:string)
        n155 = Concatenate Strings(w132, " front panel.jpg" ("string")) -> (w130:string)
        n156 = String To Path(string=w172) -> (path=w171:path)
        n157 = String To Path(string=w165) -> (path=w164:path)
        n158 = String To Path(string=w161) -> (path=w160:path)
        n159 = String To Path(string=w158) -> (path=w157:path)
        n160 = String To Path(string=w153) -> (path=w152:path)
        n161 = String To Path(string=w130) -> (path=w129:path)
        n162 = flat-sequence {
          tunnel: w173 -> [_]
          tunnel: w171 -> [w244]
          tunnel: w164 -> [w241]
          tunnel: w163 -> [w240]
          tunnel: w160 -> [w223]
          tunnel: w157 -> [w238]
          tunnel: [w227] -> w155
          tunnel: w152 -> [w217]
          tunnel: "notes updated: %b %d, %Y, %H:%M" ("time format string (%c)") -> [w216]
          tunnel: w129 -> [w212]
          frame #0 {
            n163 = local read "notes last updated"() -> (w215:timestamp)
            n164 = call "get git version.vi"() -> ("error out"=w225:errorcluster, "path to current head"=w224:path)  [unwired: 9 in, 1 out]
            n165 = Copy(8:w225, 10:w223, 11:w224) -> (0:w222:errorcluster)  [unwired: 2 in, 2 out]
            n166 = call "metadata operations.vi"("Operation"=T8."Get Spreadsheet") -> ("error out"=w243:errorcluster, "spreadsheet table"=w245:string)  [unwired: 7 in, 2 out]
            n167 = Format Date/Time String(time format string (%c)=w216, seconds (now)=w215) -> (date/time string=w221:string)  [unwired: 1 in]
            n168 = call <vilib>:"Clear Errors.vi"("error in (no error)"=w222) -> ("error out"=w226:errorcluster)  [unwired: 6 in]
            n169 = Write to Text File(file (use dialog)=w244, text=w245, error in=w243) -> (error out=w242:errorcluster)  [unwired: 1 in, 2 out]
            n170 = Write to Text File(file (use dialog)=w241, text=w240, error in=w242) -> (error out=w229:errorcluster)  [unwired: 1 in, 2 out]
            n171 = Concatenate Strings(w221, "\r\n", "notes") -> (w218:string)
            n172 = control-ref of="This VI"() -> (w213:refnum<vi>)
            n173 = call "save vi front panel image.vi"("path to JPEG file"=w212, "This VI"=w213) -> ("error out"=w211:errorcluster)  [unwired: 9 in]
            n174 = invoke class="VI" method="Ctrl Val.Get All"(reference=w213, "Controls"=TRUE) -> (error out=w237:errorcluster, "Get All Control Values Variant"=w232:cluster{"Name":string, "Variant Data":variant}[])  [unwired: 2 in, 2 out]
            n175 = Open/Create/Replace Datalog(5:w232, 8:w237, 9:enum16{"read/write", "read-only", "write-only"}."write-only" ("access (0:read/write)"), 10:T9."replace or create" ("operation (0:open)"), 11:w238) -> (0:w234:errorcluster, 3:w233:refnum<k1>)  [unwired: 1 in, 1 out]
            n176 = Write Datalog(4:w234, 6:w232, 7:w233) -> (0:w231:errorcluster, 3:w230:refnum<k1>)
            n177 = Write to Text File(file (use dialog)=w217, text=w218) -> (error out=w214:errorcluster)  [unwired: 2 in, 2 out]
            n178 = Close File(refnum=w230, error in=w231) -> (error out=w228:errorcluster)  [unwired: 1 out]
            n179 = Build Array(w229, w226, w228, w214, w211) -> (w227:errorcluster[])
          }
        }
        n180 = call "metadata operations.vi"("sw"=u32 0, "error in (no error)"=w147, "Operation"=T8."set stack writer") -> ("error out"=w146:errorcluster)  [unwired: 5 in, 3 out]
        n181 = call <vilib>:"Clear Errors.vi"("error in (no error)"=w146) -> ("error out"=w143:errorcluster)  [unwired: 6 in]
        n182 = call "stop Recording.vi"("error in (no error)"=w143, "sw"=w150) -> ("error out"=w170:errorcluster, "sw out"=w168:u32)  [unwired: 7 in, 1 out]
        n183 = call "flag experiment state.vi"("error in (no error)"=w143, "experiment started"=FALSE) -> ("error out"=w141:errorcluster)  [unwired: 9 in]
        n184 = call "get Timing Report.vi"("error in (no error)"=w170, "maxchars"=65536, "sw"=w168) -> ("error out"=w169:errorcluster, "dst"=w163:string)  [unwired: 6 in, 1 out]
        "timing report" <- w163
        n185 = call "destroy Stack Writer.vi"("error in (no error)"=w169, "sw"=w168) -> ("error out"=w184:errorcluster)  [unwired: 9 in]
        n186 = Merge Errors(w147, w184, w141) -> (w180:errorcluster)
        n187 = property on="use ROI" class="Bool (strict)"(error in=w180, "Visible"=w179) -> (error out=w176:errorcluster)  [unwired: 1 in, 1 out]
        n188 = property on="region of interest" class="Clust (strict)"(error in=w176, "Visible"=w179) -> (error out=w177:errorcluster)  [unwired: 1 in, 1 out]
        n189 = property on="STOP ACQUISITION" class="Bool"(error in=w177, "Visible"=FALSE) -> (error out=w175:errorcluster)  [unwired: 1 in, 1 out]
        n190 = Merge Errors(w175, w155) -> (w156:errorcluster)
      }
      event "set all control values as default": Mouse Up {
        # "experiment description default values bin file"
        # "vi name"
        n191 = event-data() -> ()  [unwired: 1 in, 8 out]
        n192 = control-ref of="This VI"() -> (w419:refnum<vi>)
        n193 = invoke class="VI" method="Ctrl Val.Get All"(reference=w419, error in=w418, "Controls"=TRUE) -> (error out=w410:errorcluster, "Get All Control Values Variant"=w403:cluster{"Name":string, "Variant Data":variant}[])  [unwired: 1 in, 2 out]
        n194 = Current VI's Path() -> (path=w397:path)
        n195 = call <vilib>:"Get File Extension.vi"("file"=w397) -> ("filename without extension"=w396:string)  [unwired: 7 in, 3 out]
        n196 = Strip Path(path=w397) -> (stripped path=w416:path)  [unwired: 1 out]
        n197 = Strip Path(path=w416) -> (stripped path=w415:path)  [unwired: 1 out]
        n198 = Concatenate Strings(w396, " ctl values.dflt" ("string")) -> (w411:string)
        n199 = File/Directory Info(path=w416, error in=w410) -> (directory=w414:bool, error out=w409:errorcluster)  [unwired: 5 out]
        n200 = Select(t=w416, s=w414, f=w415) -> (s? t:f=w412:path)
        n201 = Build Path(base path=w412, name or relative path=w411) -> (appended path=w408:path)
        n202 = Open/Create/Replace Datalog(5:w403, 8:w409, 9:enum16{"read/write", "read-only", "write-only"}."write-only" ("access (0:read/write)"), 10:T9."replace or create" ("operation (0:open)"), 11:w408) -> (0:w405:errorcluster, 3:w404:refnum<k1>)  [unwired: 1 in, 1 out]
        n203 = Write Datalog(4:w405, 6:w403, 7:w404) -> (0:w402:errorcluster, 3:w401:refnum<k1>)
        n204 = Close File(refnum=w401, error in=w402) -> (error out=w399:errorcluster)  [unwired: 1 out]
        n205 = Unbundle By Name(w399) -> ("status"=w398:bool)
      }
      event "STOP PROGRAM": Mouse Up {
        n206 = event-data() -> ()  [unwired: 1 in, 8 out]
      }
      event "MAKE DIRECTORIES": Mouse Up {
        n207 = event-data() -> ()  [unwired: 1 in, 8 out]
        n208 = local read "Experiment Description"() -> (w432:T2)
        n209 = call "experiment description to file name Samuel.vi"("Experiment Description"=w432) -> ("data directory with time"=w431:path, "filename"=w430:string)  [unwired: 8 in, 1 out]
        n210 = local write "filename"(w430) -> ()
        n211 = Build Path(base path="base directory", name or relative path=w431) -> (appended path=w423:path)
        n212 = local write "data directory"(w423) -> ()
        n213 = call <vilib>:"Check if File or Folder Exists.vi"("error in (no error)"=w436, "path"=w423) -> ("error out"=w434:errorcluster, "file or folder exists?"=w433:bool, "dup path"=w435:path)  [unwired: 7 in]
        n214 = case shown="False" w433 {
          tunnel: w435 -> [w442 w448]
          tunnel: w434 -> [w441 w449]
          tunnel: [w440 w447] -> w428
          tunnel: "directory already exists and is not empty" ("message") -> [_ w445]
          tunnel: [TRUE w443] -> w427
          frame False {
            n215 = Create Folder(path (use dialog)=w442, error in=w441) -> (error out=w440:errorcluster)  [unwired: 1 in, 2 out]
          }
          frame True {
            n216 = call <vilib>:"Recursive File List.vi"("error in (no error)"=w449, "Folder Path"=w448) -> ("error out"=w447:errorcluster, "Number of Files"=w446:i32)  [unwired: 5 in, 3 out]
            n217 = Greater Than 0?(x=w446) -> (x > 0?=w444:bool)
            n218 = case shown="True" w444 {
              tunnel: w445 -> [_ w450]
              frame False {
              }
              frame True {
                n219 = One Button Dialog(message=w450) -> ()  [unwired: 1 in, 1 out]
              }
            }
            n220 = Not(x=w444) -> (.not. x?=w443:bool)
          }
        }
        n221 = control-ref of="START ACQUISITION"() -> (w438:refnum<vi>)
        n222 = property class="Bool (strict)"(reference=w438, error in=w428, "Visible"=w427) -> (error out=w424:errorcluster)  [unwired: 1 out]
        n223 = Unbundle By Name(w424) -> ("status"=w425:bool)
      }
      event "notes": Value Change {
        n224 = event-data() -> ()  [unwired: 1 in, 6 out]
        n225 = Get Date/Time In Seconds() -> (seconds since 1Jan1904=→"notes last updated":timestamp)
      }
    }
    "loop iteration" <- w59
  }
  "error out" <- w16
  n226 = call <vilib>:"Clear Errors.vi"("error in (no error)"=w16) -> ("error out"=w18:errorcluster)  [unwired: 6 in]
  n227 = call "close image source.vi"("error in (no error)"=w18, "image source data"=w19) -> ("error out"=w17:errorcluster)  [unwired: 9 in]
  n228 = Merge Errors(w16, w17) -> (w15:errorcluster)
  n229 = call <vilib>:"Simple Error Handler.vi"("type of dialog (OK msg:1)"=w14, "error in (no error)"=w15) -> ()  [unwired: 3 in, 5 out]
